vi "SE FP behavior point to dock.vi"(1 "Behavior\nVelocity":dbl, 2 "Activate?":bool=TRUE, 3 "Camera Data":T2(array[cluster]), 4 "IR Sensors":T1(array[cluster])) -> (0 "Dock Array":dbl[](array[numeric]))   [LabVIEW 2014]
panel:
  out "Waveform Graph":cluster{dbl, dbl, dbl[]}(graph)
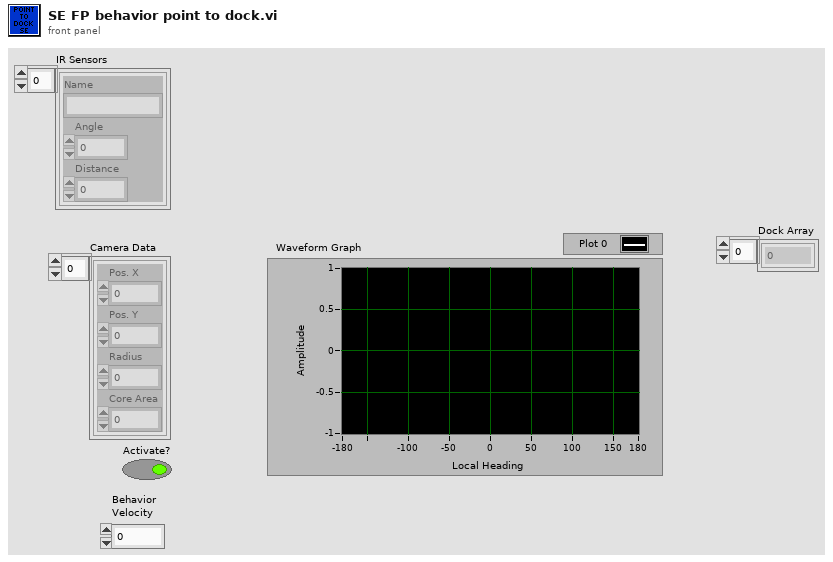
[diagram p1: front panel]
types:
  T1 = cluster{"Name":string, "Angle":dbl, "Distance":dbl}[]
  T2 = cluster{"Pos. X":i32, "Pos. Y":i32, "Radius":i32, "Core Area":i32}[]
  T3 = cluster{"Name":string, "Angle":dbl, "Distance":dbl}
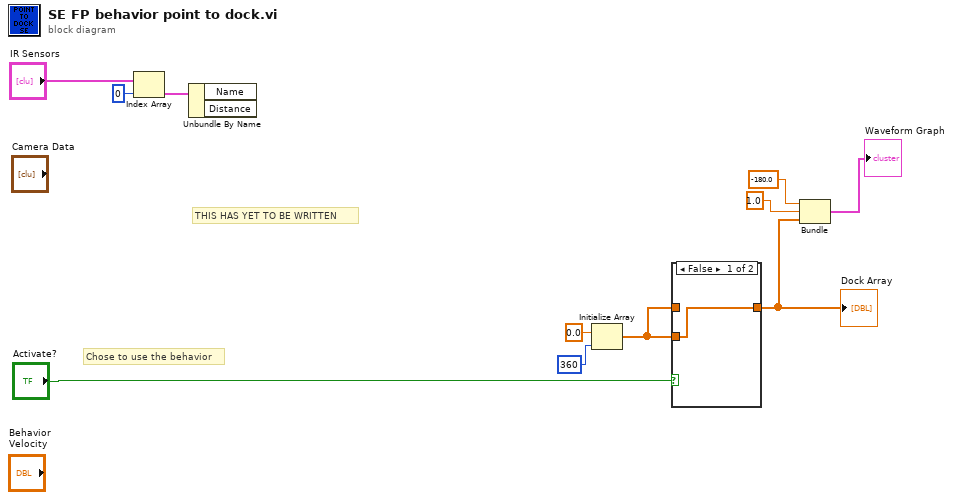
[diagram p0: block diagram]
diagram:
  # "THIS HAS YET TO BE WRITTEN"
  # "Chose to use the behavior"
  n1 = Index Array(array="IR Sensors", index=0) -> (element=w2:T3)
  n2 = Unbundle By Name(w2) -> ()  [unwired: 2 out]
  n3 = Initialize Array(0.0 ("element"), 360 ("dimension size")) -> (w5:dbl[])
  n4 = case shown="False" "Activate?" {
    tunnel: w5 -> [w12 _]
    tunnel: w5 -> [_ w13]
    tunnel: [w12 w13] -> w4
    frame False {
    }
    frame True {
    }
  }
  "Dock Array" <- w4
  n5 = Bundle(-180.0, 1.0, w4) -> (→"Waveform Graph":cluster{dbl, dbl, dbl[]})  [unwired: 1 in]
